vi "Scale_read.vi"(4 "error in (no error)":errorcluster, 7 "VISA resource name":refnum<visa-resource-name>) -> (0 "error out":errorcluster, 1 "Length of received \nmessage":i32, 2 "read buffer":string, 3 "VISA resource name out":refnum<visa-resource-name>)   [LabVIEW 2019]
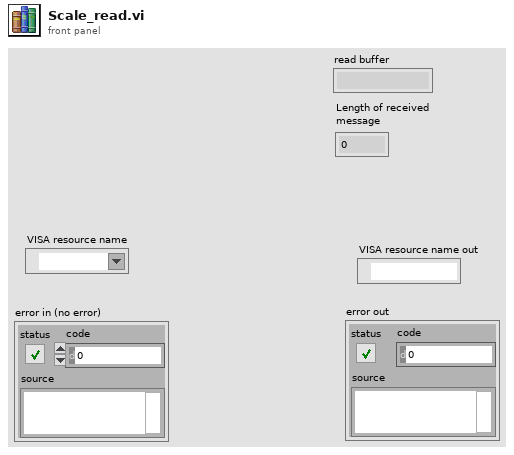
[diagram p1: front panel]
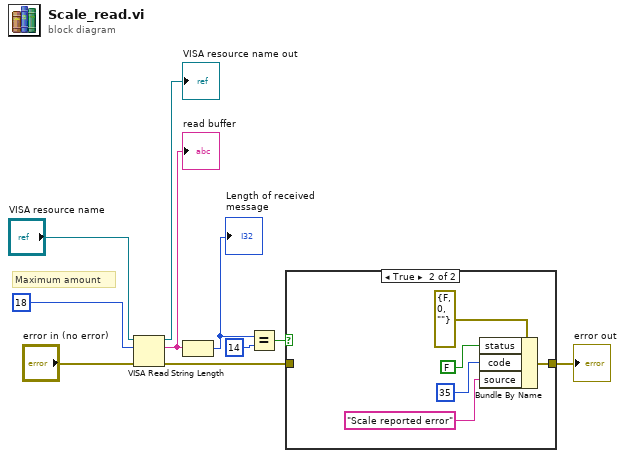
[diagram p0: block diagram]
diagram:
  # "Maximum amount"
  n1 = VISA Read(VISA resource name="VISA resource name", byte count=u32 18, error in (no error)="error in (no error)") -> (VISA resource name out=→"VISA resource name out":refnum<visa-resource-name>, read buffer=w6:string, error out=w2:errorcluster)  [unwired: 1 out]
  "read buffer" <- w6
  n2 = String Length(string=w6) -> (length=w5:i32)
  "Length of received \nmessage" <- w5
  n3 = Equal?(x=w5, y=14) -> (x = y?=w3:bool)
  n4 = case shown="True" w3 {
    tunnel: w2 -> [w11 _]
    tunnel: [w11 w15] -> w1
    frame False {
    }
    frame True {
      n5 = Bundle By Name(cluster=errorcluster {"status"=FALSE, "code"=0, "source"=""} ("error constant"), "status"=FALSE, "code"=35, "source"="Scale reported error") -> (w15:errorcluster)
    }
  }
  "error out" <- w1
